vi "FIRFilter.vi"(7 "Filter Size":dbl, 8 "Reset":bool, 11 "Input":dbl) -> (3 "Output":dbl)   [LabVIEW 2012]
panel:
  in  "Filter Strength":dbl
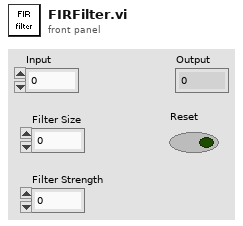
[diagram p1: front panel]
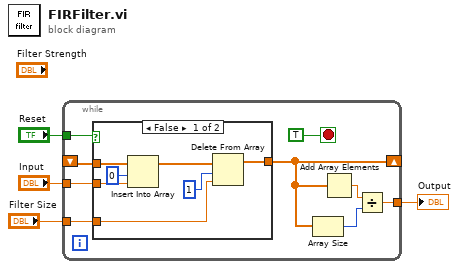
[diagram p0: block diagram]
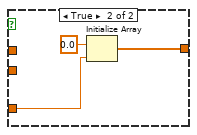
[diagram p2: hidden frame]
diagram:
  n1 = while {
    tunnel: "Reset" -> [w12]
    tunnel: "Filter Size" -> [w11]
    tunnel: "Input" -> [w9]
    shift-right: [w8] -> _
    shift-left: _ -> [w10]
    tunnel: [w5] -> w1
    stop <- TRUE stop-if-true
    n2 = case shown="False" w12 {
      tunnel: w11 -> [w19 w22]
      tunnel: w10 -> [w17 _]
      tunnel: w9 -> [w16 _]
      tunnel: [w15 w21] -> w8
      frame False {
        n3 = Insert Into Array(array=w17, index=0, new element=w16) -> (w20:dbl[])
        n4 = Delete From Array(array=w20, length=1, index=w19) -> (array with subset deleted=w15:dbl[])  [unwired: 1 out]
      }
      frame True {
        n5 = Initialize Array(0.0 ("element"), w22) -> (w21:dbl[])
      }
    }
    n6 = Array Size(array=w8) -> (size(s)=w7:i32)
    n7 = Add Array Elements(numeric array=w8) -> (sum=w6:dbl)
    n8 = Divide(x=w6, y=w7) -> (x/y=w5:dbl)
  }
  "Output" <- w1
